vi "RecupCommand.vi"(11 "Rubix initialisé via caméra":u16[][](array[numeric])=[[1, 5, 2, 4, 3, 5, 4, 2, 3], [0, 5, 4, 1, 2, 0, 5, 2, 2], [1, 2, 1, 1, 0, 0, 4, 1, 4], [3, 4, 0, 4, 1, 1, 2, 4, 3], [5, 3, 0, 2, 5, 3, 5, 0, 5], [1, 5, 2, 3, 4, 0, 0, 3, 3]]) -> (3 "Commands to Execute":string[](array[string]))   [LabVIEW 2019]
doc: "Generate a tab of command (strings) from a tab of numbers"
uses:
  Projet final 1.1/Rubik's Solver.dll
panel:
  out "Loesung":i32[](array[numeric])
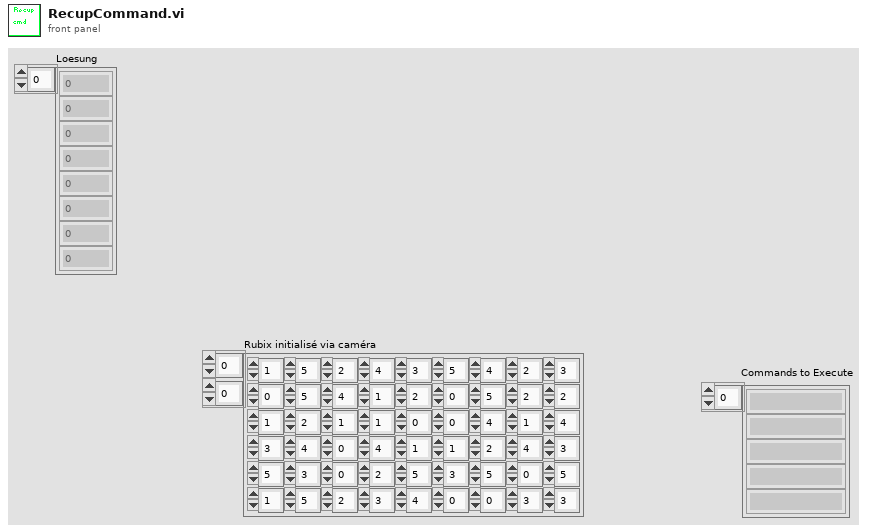
[diagram p1: front panel]
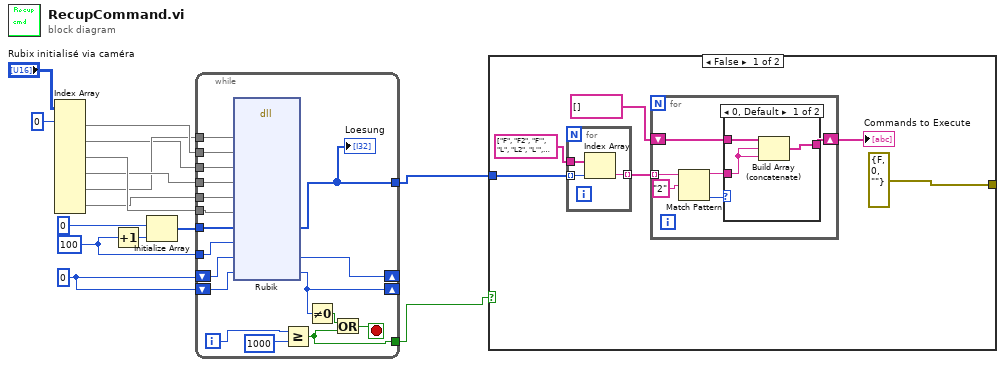
[diagram p0: block diagram]
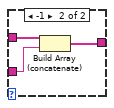
[diagram p2: hidden frame]
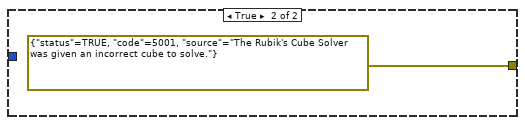
[diagram p3: hidden frame]
diagram:
  w11 = u8 0
  w12 = u16 100
  n1 = Index Array(array="Rubix initialisé via caméra", index (row) #1=0 ("disabled index (col)")) -> (element #1=w9:u16[], element #2=w4:u16[], element #3=w8:u16[], element #4=w7:u16[], element #5=w6:u16[], element #6=w5:u16[])  [unwired: 11 in]
  n2 = Increment(x=w12) -> (x+1=w14:u16)
  n3 = Initialize Array(0 ("element"), w14) -> (w13:i32[])
  n4 = while {
    tunnel: w13 -> [w33]
    shift-right: [w29] -> _
    shift-left: w11 -> [w32]
    tunnel: w12 -> [w28]
    shift-right: [w30] -> _
    shift-left: w11 -> [w31]
    tunnel: [w21] -> w2
    tunnel: w6 -> [w27]
    tunnel: w9 -> [w26]
    tunnel: w4 -> [w25]
    tunnel: w7 -> [w24]
    tunnel: w5 -> [w23]
    tunnel: w8 -> [w22]
    tunnel: [w16] -> w1
    i -> [w20]
    stop <- w17 stop-if-true
    n5 = dll-call lib="X:/Projet S8/Projet final 1.1/Rubik's Solver.dll" fn="Rubik"("Up"=w27, "Front"=w26, "Right"=w25, "Left"=w24, "Down"=w23, "Back"=w22, "Loesung"=w33, "Anzahl"=w28, "Error"=w31, "ready"=w32) -> ("Loesung"=w21:i32[], "Error"=w30:u8, "ready"=w29:u8)  [unwired: 11 in, 2 out]
    "Loesung" <- w21
    n6 = Greater Or Equal?(x=w20, y=1000 ("x")) -> (x >= y?=w16:bool)
    n7 = Not Equal To 0?(x=w29) -> (x != 0?=w18:bool)
    n8 = Or(x=w18, y=w16) -> (x .or. y?=w17:bool)
  }
  n9 = case shown="False" w1 {
    tunnel: w2 -> [w37 _]
    tunnel: [errorcluster {"status"=FALSE, "code"=0, "source"=""} ("error IO") errorcluster {"status"=TRUE, "code"=5001, "source"="The Rubik's Cube Solver  was given an incorrect cube to solve."} ("error IO")] -> _
    frame False {
      n10 = for {
        tunnel: w37 -> [w54] mode=indexing
        tunnel: [w53] -> w39 mode=indexing
        tunnel: string[] ["F", "F2", "F'", "L", "L2", "L'", "U", "U2", "U'", "B", "B2", "B'", "R", "R2", "R'", "D", "D2", "D'"] -> [w52]
        n11 = Index Array(array=w52, index=w54) -> (element=w53:string)
      }
      n12 = for {
        tunnel: w39 -> [w45] mode=indexing
        shift-right: [w40] -> w34
        shift-left: string[] [] -> [w41]
        n13 = Match Pattern(string=w45, regular expression="2") -> (before substring=w42:string, offset past match=w43:i32)  [unwired: 1 in, 2 out]
        n14 = case shown="0, Default" w43 {
          tunnel: w42 -> [w46 w49]
          tunnel: w41 -> [w48 w51]
          tunnel: [w47 w50] -> w40
          frame 0, Default {
            n15 = Build Array (concatenate)(w48, w46, w46) -> (w47:string[])
          }
          frame -1 {
            n16 = Build Array (concatenate)(w51, w49) -> (w50:string[])
          }
        }
      }
      "Commands to Execute" <- w34
    }
    frame True {
    }
  }
